vi "TIO Serial Port Discovery.vi"(11 "Default baud":u32=115200) -> (2 "Device Names":string[](array[string])=["/dev/cu.Bluetooth-Incoming-Port", "", "/dev/cu.usbserial-00000"], 3 "VISA Names":string[](array[string])=["ASRL1::INSTR", "ASRL2::INSTR", "ASRL3::INSTR"])   [LabVIEW 2010]
uses:
  <vilib>/Instr/_visa.llb/VISA Open Access Mode.ctl
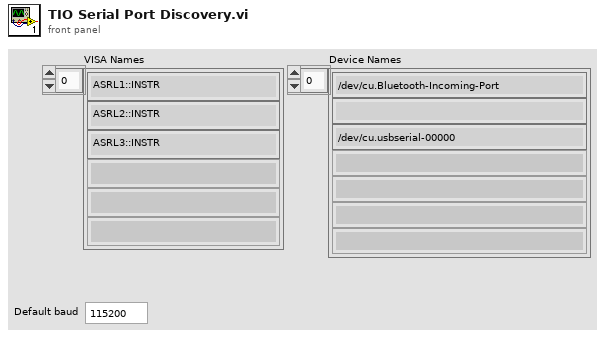
[diagram p1: front panel]
types:
  T1 = typedef "VISA Open Access Mode.ctl" = u32
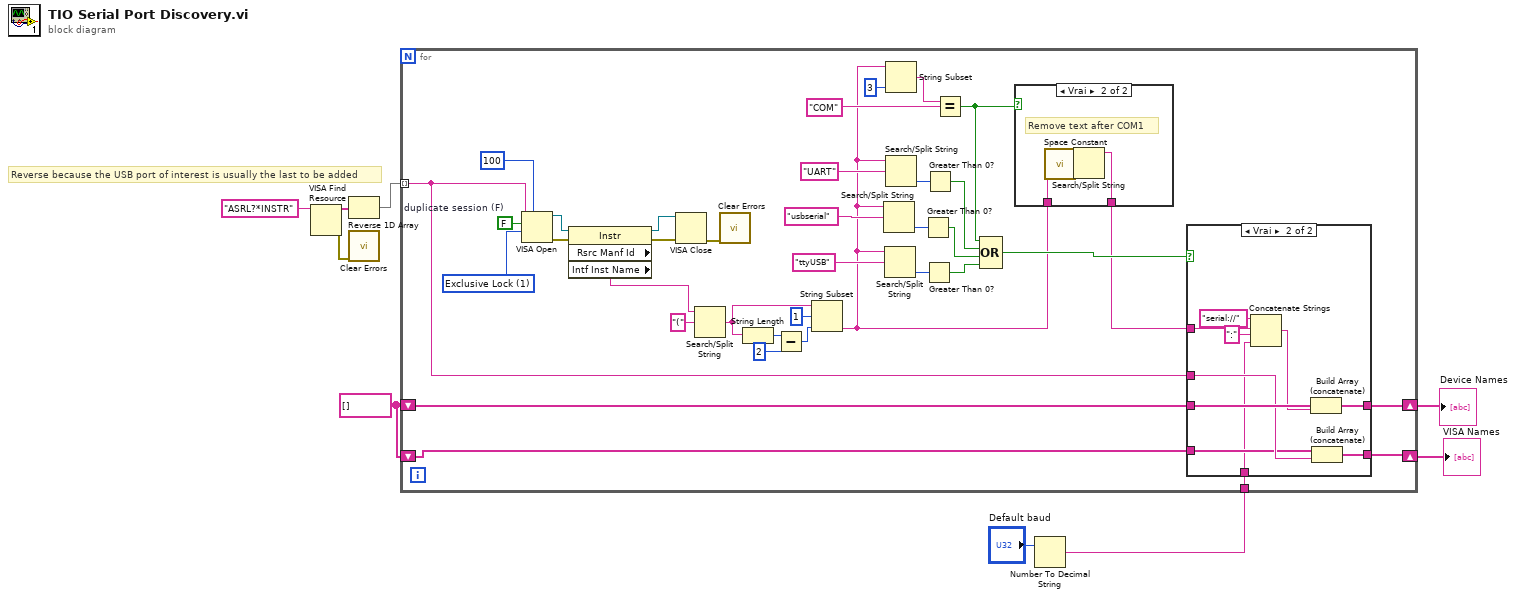
[diagram p0: block diagram]
diagram:
  w7 = string[] []
  # "Reverse because the USB port of interest is usually the last to be added"
  n1 = VISA Find Resource(11:"ASRL?*INSTR" ("expression (\"?*\")")) -> (0:w1:errorcluster, 3:w3:string[])  [unwired: 2 in, 1 out]
  n2 = Reverse 1D Array(array=w3) -> (reversed array=w2:string[])
  n3 = call <vilib>:"Clear Errors.vi"("error in (no error)"=w1) -> ()  [unwired: 6 in, 1 out]
  n4 = Number To Decimal String(number="Default baud") -> (decimal integer string=w4:string)  [unwired: 1 in]
  n5 = for {
    tunnel: w2 -> [w31] mode=indexing
    shift-right: [w43] -> w8
    shift-left: w7 -> [w32]
    shift-right: [w29] -> w6
    shift-left: w7 -> [w30]
    tunnel: w4 -> [w17]
    w11 = T1 1 items=["VISA Defaults"=0, "Exclusive Lock"=1, "Load Configured Settings"=4] ("Access Mode")
    w45 = FALSE  # duplicate session (F)
    n6 = VISA Open(timeout (0)=u32 100 ("VISA Open timeout (0)"), duplicate session (F)=w45, access mode=w11, VISA resource name=w31) -> (VISA resource name=w46:refnum<visa-resource-name>, error out=w44:errorcluster)  [unwired: 1 in]
    n7 = property class="Instr" props=["Rsrc Manf Id", "Intf Inst Name"](reference=w46, error in=w44) -> (reference out=w35:refnum<visa-resource-name>, error out=w34:errorcluster, "Intf Inst Name"=w36:string)  [unwired: 1 out]
    n8 = VISA Close(VISA resource name=w35, error in (no error)=w34) -> (error out=w33:errorcluster)
    n9 = Search/Split String(string=w36, search string/char (-)="(") -> (match + rest of string=w38:string)  [unwired: 1 in, 2 out]
    n10 = call <vilib>:"Clear Errors.vi"("error in (no error)"=w33) -> ()  [unwired: 6 in, 1 out]
    n11 = String Length(string=w38) -> (length=w40:i32)
    n12 = Subtract(x=w40, y=2) -> (x-y=w41:i32)
    n13 = String Subset(string=w38, offset (0)=1, length (rest)=w41) -> (substring=w12:string)
    n14 = Search/Split String(string=w12, search string/char (-)="usbserial") -> (offset of match=w27:i32)  [unwired: 1 in, 2 out]
    n15 = Search/Split String(string=w12, search string/char (-)="ttyUSB") -> (offset of match=w26:i32)  [unwired: 1 in, 2 out]
    n16 = String Subset(string=w12, length (rest)=3 ("length (rest)")) -> (substring=w19:string)  [unwired: 1 in]
    n17 = Search/Split String(string=w12, search string/char (-)="UART") -> (offset of match=w14:i32)  [unwired: 1 in, 2 out]
    n18 = Greater Than 0?(x=w27) -> (x > 0?=w23:bool)
    n19 = Greater Than 0?(x=w26) -> (x > 0?=w24:bool)
    n20 = Greater Than 0?(x=w14) -> (x > 0?=w21:bool)
    n21 = Equal?(x=w19, y="COM" ("search string/char (-)")) -> (x = y?=w16:bool)
    n22 = Compound Arithmetic op=OR(w16, w21, w23, w24) -> (w22:bool)
    n23 = case shown="Vrai" w16 {
      tunnel: w12 -> [w47 w49]
      tunnel: [w47 w48] -> w15
      frame False {
      }
      frame True {
        # "Remove text after COM1"
        n24 = call <vilib>:"Space Constant.vi"() -> ("String"=w50:string)
        n25 = Search/Split String(string=w49, search string/char (-)=w50) -> (substring before match=w48:string)  [unwired: 1 in, 2 out]
      }
    }
    n26 = case shown="Vrai" w22 {
      tunnel: [w52 w62] -> w43
      tunnel: w15 -> [_ w57]
      tunnel: w32 -> [w52 w61]
      tunnel: w31 -> [_ w60]
      tunnel: w30 -> [w51 w59]
      tunnel: [w51 w58] -> w29
      tunnel: w17 -> [_ w53]
      frame False {
      }
      frame True {
        n27 = Concatenate Strings("serial://" ("string"), w57, ":" ("string"), w53) -> (w56:string)
        n28 = Build Array (concatenate)(w61, w56) -> (w62:string[])
        n29 = Build Array (concatenate)(w59, w60) -> (w58:string[])
      }
    }
  }
  "VISA Names" <- w6
  "Device Names" <- w8
